vi "Facade.vi"(0 "Data In":T37={"Waveform"={"Type"=enum."Tone", "Tone"={"Frequency (kHz)"=0.0, "Phase (cycles)"=0.0, "Random phase"=FALSE}, "Pulse Train"={"Pulse width (us)"=0.0, "Pulse rate (Hz)"=0.0, "Gap (ms)"=0.0, "Polarity"=enum."POS", "PT State"={"Template"=[], "Nperiod"=0, "Index"=0, "Pulse Rate (Hz)"=0.0, "Phase (cycles)"=0.0, "Noff"=0}, "Asynch"=FALSE}, "Noise"={"Properties"={"InvFilt"=FALSE, "Aweight"=FALSE, "Seed"=0, "Tokens"=0, "Brickwall"=FALSE}, "Data"={"TokenNum"=0}}, "File"={"Filename"=path "", "Signal"=[], "Channel"=0, "stream"=FALSE, "offset"=0, "nreps"=0, "loops"=0, "Randomize"=FALSE, "order"=[], "Seed"=0, "Tokens"=0}, "FMSweep"={"Rate (oct/s)"=0.0, "Fmin (Hz)"=0.0, "Fmax (Hz)"=0.0, "Ramp (ms)"=0.0, "Linear"=FALSE}, "Chirp Train"={"Params"={"Fmin (kHz)"=4.0, "Fmax (kHz)"=64.0, "Compensate"=FALSE, "Duration (ms)"=2.0}, "Data"={"WF"=[]}}, "Complex Tone"={"Params"={"F0 (Hz)"=0.0, "Band"={"Flow (Hz)"=0.0, "Fhigh (Hz)"=0.0}, "Phase"=enum."Cosine", "Min F0 (Hz)"=0.0, "Max F0 (Hz)"=0.0, "ContinRandPhase"=FALSE, "Max peak factor"=inf, "Max mod depth"=2.0, "MinHarmNum"=0, "MaxHarmNum"=0, "Level Mode"=enum."per component", "% jitter"=0.0}, "Data"={"Ncomp"=0, "MinHarm"=0, "Phase"=[], "Amplitude"=[], "Npts/frame"=0, "Last F0"=0.0, "Fmin"=0.0, "Fmax"=0.0, "Lslope"=0.0, "randphase"=FALSE, "overall rms"=FALSE, "fmult"=[], "jittered"=FALSE}}, "FM"={"Carrier (kHz)"=0.0, "ModRate (Hz)"=0.0, "Depth (Hz)"=0.0, "Phase (cycles)"=0.0}, "Vowel"={"Freqs"="", "Set level"=enum."Total", "Freq"=[], "weights"=[]}, "Ramp"={"Duration (ms)"=0.0}}, "Filter"={"Type"=enum."Lowpass", "CF (kHz)"=0.0, "BW (kHz)"=0.0, "Cascade"=FALSE, "Quadrature"=FALSE, "Scale Factor"=0.0, "Stages"=[], "Class"=enum."Elliptic", "Order"=0, "BWUnits"=enum."Linear"}, "Burst"={"Active"=FALSE, "Delay (ms)"=0.0, "Duration (ms)"=50.0, "Ramp (ms)"=5.0, "Rate (Hz)"=0.0, "Trepeat (ms)"=0.0, "Repeat"=FALSE}, "Level"={"Level"=0.0, "Units"=enum."dB atten", "Max"=0.0, "Data"={"Multiplier"=0.0, "Cal File"=path "", "Cal"={"Freq (Hz)"=[], "Mag (dB SPL)"=[], "Phase (deg)"=[]}, "audiogram"=path ""}}, "Name"="", "Advanced"={"AltPol"=FALSE, "Var"="", "Expr"=""}, "SAM"={"Active"=FALSE, "Frequency (Hz)"=0.0, "Depth"=0.0, "Init Phase (cycles)"=0.0, "phase (degrees)"=0.0, "Asynch"=FALSE}, "Destination"={"Name"="", "Num"=0}} {"Filter"."Stages"."IIR Filter"."Forward Coefficients" format="%.4f"; "Filter"."Stages"."IIR Filter"."Reverse Coefficients" format="%.4f"}, 2 "Display State In":T29, 3 "Container State":T36) -> (6 "Data Out":T37={"Waveform"={"Type"=enum."Tone", "Tone"={"Frequency (kHz)"=0.0, "Phase (cycles)"=0.0, "Random phase"=FALSE}, "Pulse Train"={"Pulse width (us)"=0.0, "Pulse rate (Hz)"=0.0, "Gap (ms)"=0.0, "Polarity"=enum."POS", "PT State"={"Template"=[], "Nperiod"=0, "Index"=0, "Pulse Rate (Hz)"=0.0, "Phase (cycles)"=0.0, "Noff"=0}, "Asynch"=FALSE}, "Noise"={"Properties"={"InvFilt"=FALSE, "Aweight"=FALSE, "Seed"=0, "Tokens"=0, "Brickwall"=FALSE}, "Data"={"TokenNum"=0}}, "File"={"Filename"=path "", "Signal"=[], "Channel"=0, "stream"=FALSE, "offset"=0, "nreps"=0, "loops"=0, "Randomize"=FALSE, "order"=[], "Seed"=0, "Tokens"=0}, "FMSweep"={"Rate (oct/s)"=0.0, "Fmin (Hz)"=0.0, "Fmax (Hz)"=0.0, "Ramp (ms)"=0.0, "Linear"=FALSE}, "Chirp Train"={"Params"={"Fmin (kHz)"=4.0, "Fmax (kHz)"=64.0, "Compensate"=FALSE, "Duration (ms)"=2.0}, "Data"={"WF"=[]}}, "Complex Tone"={"Params"={"F0 (Hz)"=0.0, "Band"={"Flow (Hz)"=0.0, "Fhigh (Hz)"=0.0}, "Phase"=enum."Cosine", "Min F0 (Hz)"=0.0, "Max F0 (Hz)"=0.0, "ContinRandPhase"=FALSE, "Max peak factor"=inf, "Max mod depth"=2.0, "MinHarmNum"=0, "MaxHarmNum"=0, "Level Mode"=enum."per component", "% jitter"=0.0}, "Data"={"Ncomp"=0, "MinHarm"=0, "Phase"=[], "Amplitude"=[], "Npts/frame"=0, "Last F0"=0.0, "Fmin"=0.0, "Fmax"=0.0, "Lslope"=0.0, "randphase"=FALSE, "overall rms"=FALSE, "fmult"=[], "jittered"=FALSE}}, "FM"={"Carrier (kHz)"=0.0, "ModRate (Hz)"=0.0, "Depth (Hz)"=0.0, "Phase (cycles)"=0.0}, "Vowel"={"Freqs"="", "Set level"=enum."Total", "Freq"=[], "weights"=[]}, "Ramp"={"Duration (ms)"=0.0}}, "Filter"={"Type"=enum."Lowpass", "CF (kHz)"=0.0, "BW (kHz)"=0.0, "Cascade"=FALSE, "Quadrature"=FALSE, "Scale Factor"=0.0, "Stages"=[], "Class"=enum."Elliptic", "Order"=0, "BWUnits"=enum."Linear"}, "Burst"={"Active"=FALSE, "Delay (ms)"=0.0, "Duration (ms)"=50.0, "Ramp (ms)"=5.0, "Rate (Hz)"=0.0, "Trepeat (ms)"=0.0, "Repeat"=FALSE}, "Level"={"Level"=0.0, "Units"=enum."dB atten", "Max"=0.0, "Data"={"Multiplier"=0.0, "Cal File"=path "", "Cal"={"Freq (Hz)"=[], "Mag (dB SPL)"=[], "Phase (deg)"=[]}, "audiogram"=path ""}}, "Name"="", "Advanced"={"AltPol"=FALSE, "Var"="", "Expr"=""}, "SAM"={"Active"=FALSE, "Frequency (Hz)"=0.0, "Depth"=0.0, "Init Phase (cycles)"=0.0, "phase (degrees)"=0.0, "Asynch"=FALSE}, "Destination"={"Name"="", "Num"=0}} {"Filter"."Stages"."IIR Filter"."Forward Coefficients" format="%.4f"; "Filter"."Stages"."IIR Filter"."Reverse Coefficients" format="%.4f"}, 7 "Display State Out":T29, 8 "Action":T28)   [LabVIEW 2020, in "Stimulus Channel (G3).xctl"]
uses:
  Stimulus Channel (G3).xctl
  Full Stimulus Channel Data.ctl
  Waveform XControls/Waveform (G3)/Waveform Data.ctl
  Waveform VIs/Waveform Enum (V3).ctl
  Waveform XControls/Tone (G3)/Tone.Properties.ctl
  Waveform VIs/Pulse Train VIs/Pulse Train Params.ctl
  Waveform VIs/Pulse Train VIs/Pulse Polarity.ctl
  Waveform VIs/Pulse Train VIs/PT-Continuous State.ctl
  Waveform VIs/Noise VIs/Noise (G3).ctl
  Waveform VIs/Noise VIs/Noise (G3).Properties.ctl
  Waveform VIs/Noise VIs/Noise (G3).Data.ctl
  Waveform VIs/File VIs/StimFile-Params.ctl
  Waveform VIs/FM Sweep VIs/FM Sweep Params.ctl
  Waveform VIs/Chirp Train VIs/Chirp Train.ctl
  Waveform VIs/Chirp Train VIs/Chirp Train Params.ctl
  Waveform VIs/Complex Tone VIs/CT-Params.ctl
  Waveform VIs/Complex Tone VIs/CT-Phase Enum.ctl
  Waveform VIs/Complex Tone VIs/CT-Runtime Data.ctl
  Waveform XControls/FM Tone/Data.ctl
  Waveform XControls/Vowel/Vowel.Properties.ctl
  Waveform VIs/Ramp VIs/Ramp.Properties.ctl
  Filter (G3)/Filter Data.ctl
  Filter (G3)/Filter Type.ctl
  Filter VIs/Filter-Bandwidth Units.ctl
  Controls/Burst XCtl/Burst Data.ctl
  Level (G3)/Level Data.ctl
  Level (G3)/Level Units (G3).ctl
  Advanced Options (G3)/Advanced Options (G3).ctl
  Modulation VIs/SAM VIs/SAM Params.ctl
  Typedefs/Destination.ctl
  <vilib>/_xctls/Container State.ctl
  State.ctl
  Burst (G3)/Controls.ctl
  Waveform XControls/Waveform (G3)/Waveform (G3).xctl
  Level (G3)/Level (G3).xctl
  Utility VIs/Controls/KRing/KRing.xctl
  Burst (G3)/Burst (G3).xctl
  Waveform XControls/Waveform (G3)/Waveform (G3) - Persistent.ctl
  Waveform XControls/Noise (G3)/Noise (G3) - Persistent.ctl
  Calibration VIs/Endpoint VIs/LV Source/Endpoint-Spec.ctl
  Calibration VIs/Endpoint VIs/LV Source/Endpoint-Modality.ctl
  Calibration VIs/Endpoint VIs/LV Source/Endpoint-Laterality.ctl
  <vilib>/_xctls/Action.ctl
  Filter (G3)/Filter (G3).xctl
  Advanced Options (G3)/Advanced Options (G3).xctl
  <vilib>/_xctls/XControlSupport.lvlib
  Controls/Burst XCtl/Burst Control.xctl
  Waveform XControls/Noise (G3)/Noise (G3).xctl
  Waveform XControls/Tone (G3)/Tone (G3).xctl
  Waveform XControls/FM Tone/FM Tone.xctl
  Waveform XControls/Vowel/Vowel.xctl
panel:
  in  "display state signal":bool
  in  "Level Tab":enum32{"Level"}(tab)
  in  "Level":T2(xcontrol)
  in  "Tab Control 2":enum32{"Waveform"}(tab)
  in  "Waveform (G3)":T21(xcontrol)
  in  "Name":string
  in  "Destination":i16(xcontrol)
  in  "Tab Control":enum32{"Gate", "Modulation", "Filter", "More"}(tab)
  in  "Gate":T22(xcontrol)
  in  "SAM":T23
  in  "Filter":T26(xcontrol)
  in  "Advanced":T27(xcontrol)
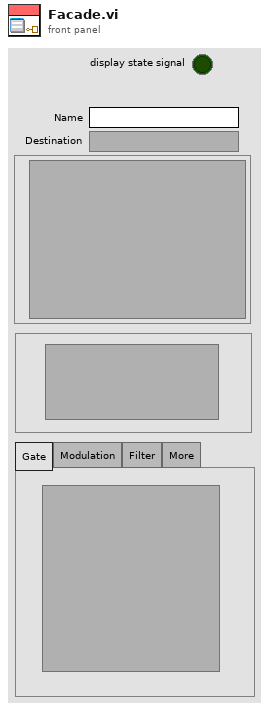
[diagram p1: front panel]
types:
  T1 = typedef "Level (G3).xctl/Level Units (G3).ctl" = enum16{"dB atten", "dB SPL", "dB re 1 Vrms", "dB V/Hz½", "mW", "dB HL", "Volts", "dB mW"}
  T2 = cluster{"Level":dbl, "Units":T1, "Max":dbl, "Data":cluster{"Multiplier":dbl, "Cal File":path, "Cal":cluster{"Freq (Hz)":dbl[], "Mag (dB SPL)":dbl[], "Phase (deg)":dbl[]}, "audiogram":path}}
  T3 = typedef "Waveform Enum (V3).ctl" = enum16{"OFF", "Tone", "Noise", "Pulse Train", "File", "FM Sweep", "Chirp Train", "Complex Tone", "FM Tone", "Vowel", "Ramp"}
  T4 = typedef "Tone (G3).xctl/Tone.Properties.ctl" = cluster{"Frequency (kHz)":dbl, "Phase (cycles)":dbl, "Random phase":bool}
  T5 = typedef "Pulse Train Params.ctl" = cluster{"Pulse width (us)":dbl, "Pulse rate (Hz)":dbl, "Gap (ms)":dbl, "Polarity":T6, "PT State":T7, "Asynch":bool}
  T6 = typedef "Pulse Polarity.ctl" = enum16{"POS", "NEG", "POS-NEG", "NEG-POS"}
  T7 = typedef "PT-Continuous State.ctl" = cluster{"Template":dbl[], "Nperiod":i32, "Index":i32, "Pulse Rate (Hz)":dbl, "Phase (cycles)":dbl, "Noff":i32}
  T8 = typedef "Noise (G3).ctl" = cluster{"Properties":T9, "Data":T10}
  T9 = typedef "Noise (G3).Properties.ctl" = cluster{"InvFilt":bool, "Aweight":bool, "Seed":i32, "Tokens":i32, "Brickwall":bool}
  T10 = typedef "Noise (G3).Data.ctl" = cluster{"TokenNum":i32}
  T11 = typedef "StimFile-Params.ctl" = cluster{"Filename":path, "Signal":dbl[], "Channel":i32, "stream":bool, "offset":i32, "nreps":i32, "loops":i32, "Randomize":bool, "order":i32[], "Seed":i32, "Tokens":i32}
  T12 = typedef "FM Sweep Params.ctl" = cluster{"Rate (oct/s)":dbl, "Fmin (Hz)":dbl, "Fmax (Hz)":dbl, "Ramp (ms)":dbl, "Linear":bool}
  T13 = typedef "Chirp Train.ctl" = cluster{"Params":T14, "Data":cluster{"WF":dbl[]}}
  T14 = typedef "Chirp Train Params.ctl" = cluster{"Fmin (kHz)":dbl, "Fmax (kHz)":dbl, "Compensate":bool, "Duration (ms)":dbl}
  T15 = typedef "CT-Params.ctl" = cluster{"F0 (Hz)":dbl, "Band":cluster{"Flow (Hz)":dbl, "Fhigh (Hz)":dbl}, "Phase":T16, "Min F0 (Hz)":dbl, "Max F0 (Hz)":dbl, "ContinRandPhase":bool, "Max peak factor":dbl, "Max mod depth":dbl, "MinHarmNum":i32, "MaxHarmNum":i32, "Level Mode":enum16{"per component", "overall rms"}, "% jitter":dbl}
  T16 = typedef "CT-Phase Enum.ctl" = enum16{"Cosine", "Random", "Alternating"}
  T17 = typedef "CT-Runtime Data.ctl" = cluster{"Ncomp":i32, "MinHarm":i32, "Phase":dbl[], "Amplitude":dbl[], "Npts/frame":i32, "Last F0":dbl, "Fmin":dbl, "Fmax":dbl, "Lslope":dbl, "randphase":bool, "overall rms":bool, "fmult":dbl[], "jittered":bool}
  T18 = typedef "FM Tone.xctl/Data.ctl" = cluster{"Carrier (kHz)":dbl, "ModRate (Hz)":dbl, "Depth (Hz)":dbl, "Phase (cycles)":dbl}
  T19 = typedef "Vowel.xctl/Vowel.Properties.ctl" = cluster{"Freqs":string, "Set level":enum16{"Total", "Per component"}, "Freq":dbl[], "weights":dbl[]}
  T20 = typedef "Ramp.Properties.ctl" = cluster{"Duration (ms)":dbl}
  T21 = cluster{"Type":T3, "Tone":T4, "Pulse Train":T5, "Noise":T8, "File":T11, "FMSweep":T12, "Chirp Train":T13, "Complex Tone":cluster{"Params":T15, "Data":T17}, "FM":T18, "Vowel":T19, "Ramp":T20}
  T22 = cluster{"Active":bool, "Delay (ms)":dbl, "Duration (ms)":dbl, "Ramp (ms)":dbl, "Rate (Hz)":dbl, "Trepeat (ms)":dbl, "Repeat":bool}
  T23 = cluster{"Active":bool, "Frequency (Hz)":dbl, "Depth (0-1)":dbl, "Phase (cycles)":dbl, "phase":dbl, "Asynch":bool}
  T24 = typedef "Filter (G3).xctl/Filter Type.ctl" = enum16{"OFF", "Lowpass", "Highpass", "Bandpass", "Bandstop"}
  T25 = typedef "Filter-Bandwidth Units.ctl" = enum16{"Linear", "Octaves", "Min-Max"}
  T26 = cluster{"Type":T24, "CF (kHz)":dbl, "BW (kHz)":dbl, "Cascade":bool, "Quadrature":bool, "Scale Factor":dbl, "Stages":cluster{"IIR Filter":cluster{"filter structure":enum32{"IIR 2nd Order", "IIR 4th Order"}, "Reverse Coefficients":dbl[], "Forward Coefficients":dbl[]}, "State":dbl[]}[], "Class":enum16{"Elliptic", "Butterworth"}, "Order":i32, "BWUnits":T25}
  T27 = cluster{"AltPol":bool, "Var":string, "Expr":string}
  T28 = typedef "XControlSupport.lvlib/Action.ctl" = cluster{"Data Changed?":bool, "State Changed?":bool, "Action Name":string}
  T29 = typedef "Stimulus Channel (G3).xctl/State.ctl" = cluster{"Show advanced":bool, "Show rove":bool, "Show name":bool, "Show dest":bool, "Lock dest":bool, "max level":dbl, "LMax Event":refnum<user-event>, "Controls":T30, "Level units":T1[], "Waveforms":T3[], "waveform":T31, "Endpoint Config":T33[], "multi":bool}
  T30 = typedef "Controls.ctl" = cluster{"Waveform":refnum<vi>, "Level":refnum<vi>, "Dest":refnum<vi>, "Gate":refnum<vi>}
  T31 = typedef "Waveform (G3).xctl/Waveform (G3) - Persistent.ctl" = cluster{"noise":T32, "Sort":bool}
  T32 = typedef "Noise (G3).xctl/Noise (G3) - Persistent.ctl" = cluster{"Show Aweight":bool}
  T33 = typedef "Endpoint-Spec.ctl" = cluster{"Name":string, "Modality":T34, "Laterality":T35, "CalFile":path, "Audiogram":path, "reuse cal?":bool}
  T34 = typedef "Endpoint-Modality.ctl" = enum16{"Unspecified", "Acoustic", "Electric", "Optical"}
  T35 = typedef "Endpoint-Laterality.ctl" = enum16{"N/A", "Right", "Left"}
  T36 = typedef "XControlSupport.lvlib/Container State.ctl" = cluster{"Indicator?":bool, "Run Mode?":bool, " Refnum":refnum<vi>}
  T37 = typedef "Stimulus Channel (G3).xctl/Full Stimulus Channel Data.ctl" = cluster{"Waveform":T38, "Filter":T39, "Burst":T40, "Level":T41, "Name":string, "Advanced":T42, "SAM":T43, "Destination":T44}
  T38 = typedef "Waveform (G3).xctl/Waveform Data.ctl" = cluster{"Type":T3, "Tone":T4, "Pulse Train":T5, "Noise":T8, "File":T11, "FMSweep":T12, "Chirp Train":T13, "Complex Tone":cluster{"Params":T15, "Data":T17}, "FM":T18, "Vowel":T19, "Ramp":T20}
  T39 = typedef "Filter (G3).xctl/Filter Data.ctl" = cluster{"Type":T24, "CF (kHz)":dbl, "BW (kHz)":dbl, "Cascade":bool, "Quadrature":bool, "Scale Factor":dbl, "Stages":cluster{"IIR Filter":cluster{"filter structure":enum32{"IIR 2nd Order", "IIR 4th Order"}, "Reverse Coefficients":dbl[], "Forward Coefficients":dbl[]}, "State":dbl[]}[], "Class":enum16{"Elliptic", "Butterworth"}, "Order":i32, "BWUnits":T25}
  T40 = typedef "Burst Control.xctl/Burst Data.ctl" = cluster{"Active":bool, "Delay (ms)":dbl, "Duration (ms)":dbl, "Ramp (ms)":dbl, "Rate (Hz)":dbl, "Trepeat (ms)":dbl, "Repeat":bool}
  T41 = typedef "Level (G3).xctl/Level Data.ctl" = cluster{"Level":dbl, "Units":T1, "Max":dbl, "Data":cluster{"Multiplier":dbl, "Cal File":path, "Cal":cluster{"Freq (Hz)":dbl[], "Mag (dB SPL)":dbl[], "Phase (deg)":dbl[]}, "audiogram":path}}
  T42 = typedef "Advanced Options (G3).xctl/Advanced Options (G3).ctl" = cluster{"AltPol":bool, "Var":string, "Expr":string}
  T43 = typedef "SAM Params.ctl" = cluster{"Active":bool, "Frequency (Hz)":dbl, "Depth":dbl, "Init Phase (cycles)":dbl, "phase (degrees)":dbl, "Asynch":bool}
  T44 = typedef "Destination.ctl" = cluster{"Name":string, "Num":i32}
  T45 = enum8{"Enabled", "Disabled", "Disabled and Grayed Out"}
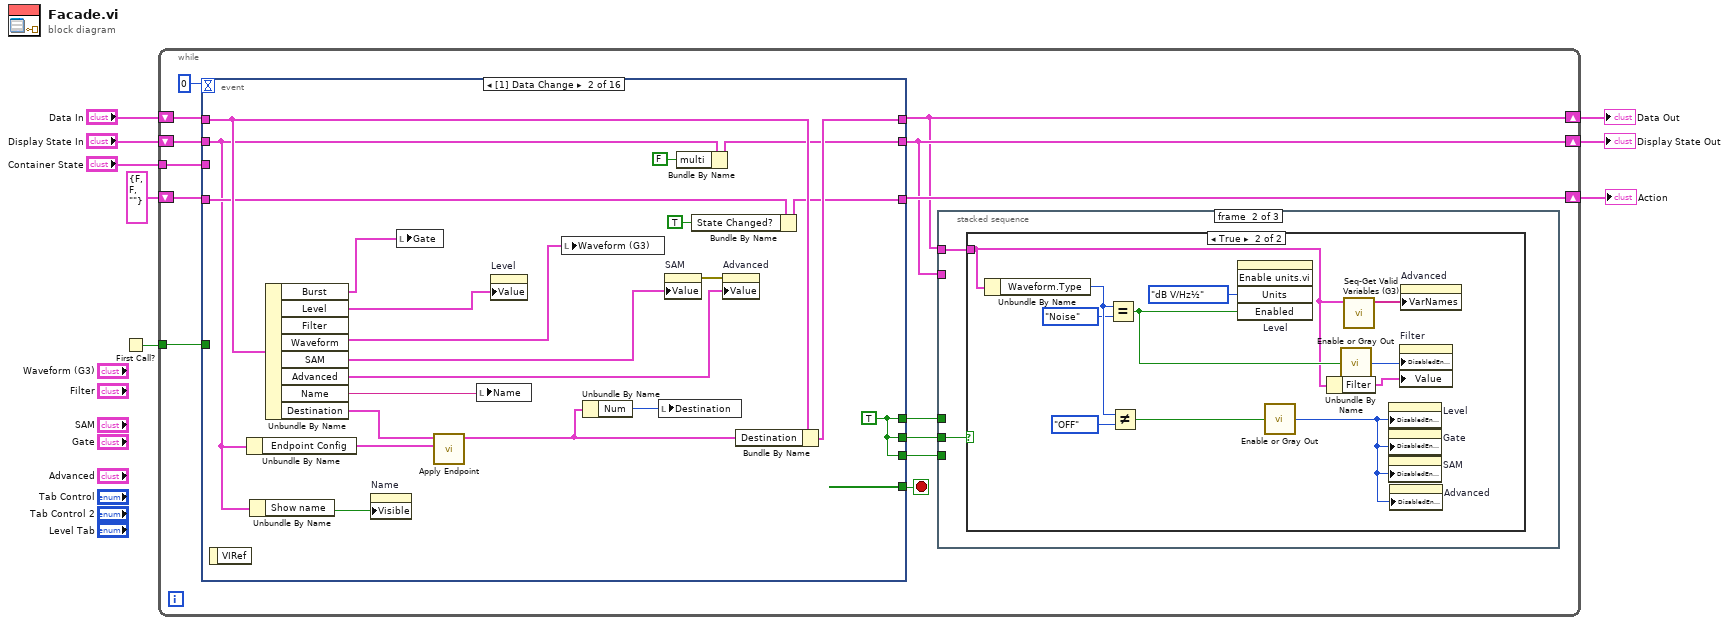
[diagram p0: block diagram]
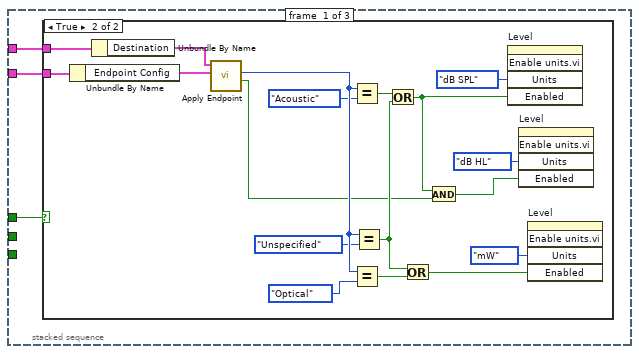
[diagram p2: hidden frame]
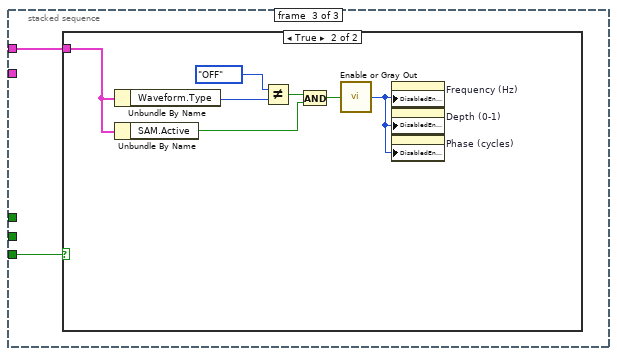
[diagram p5: hidden frame]
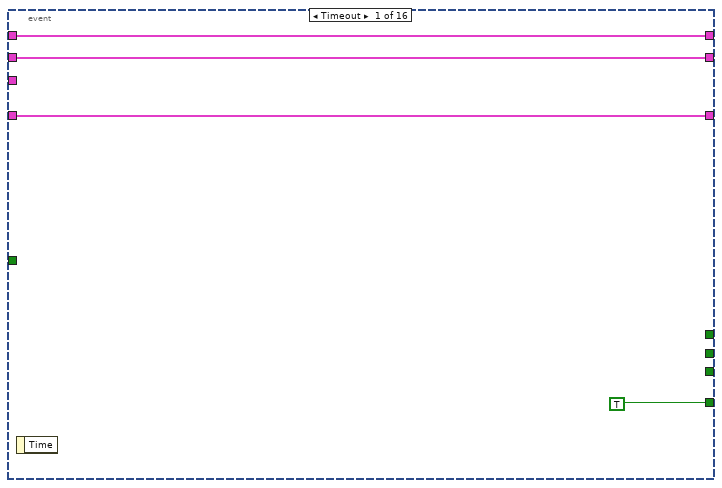
[diagram p7: hidden frame]
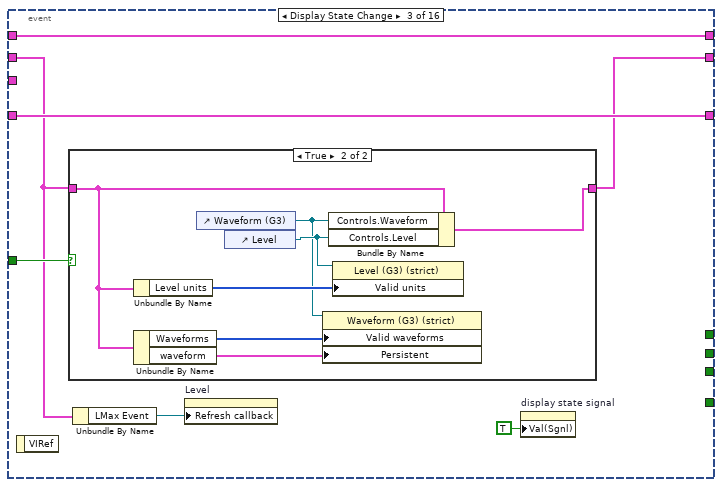
[diagram p8: hidden frame]
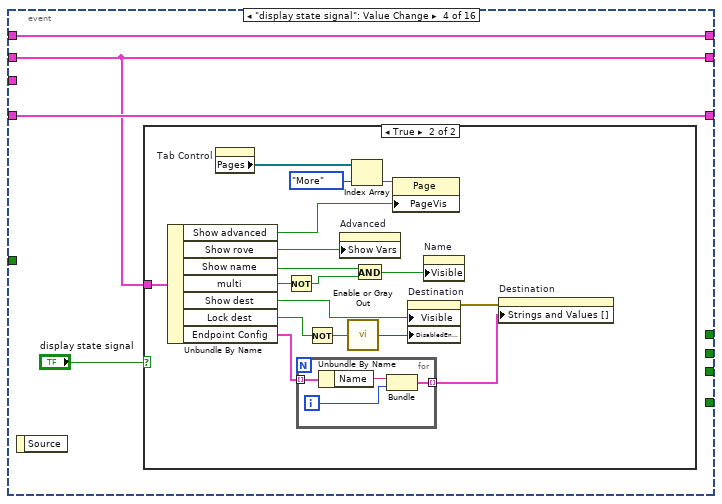
[diagram p10: hidden frame]
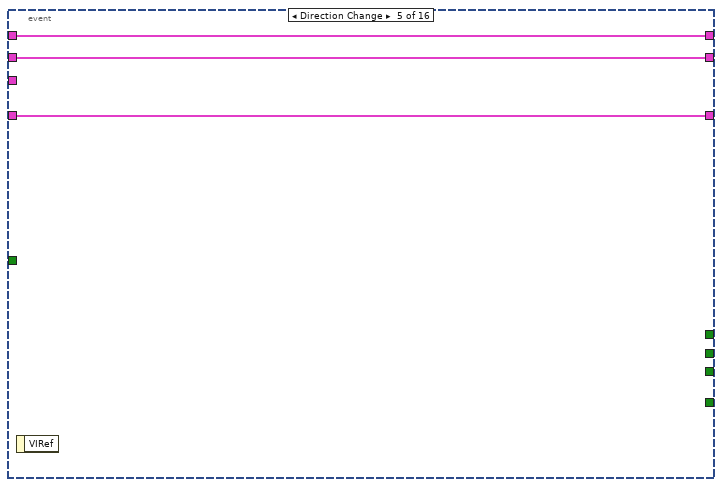
[diagram p12: hidden frame]
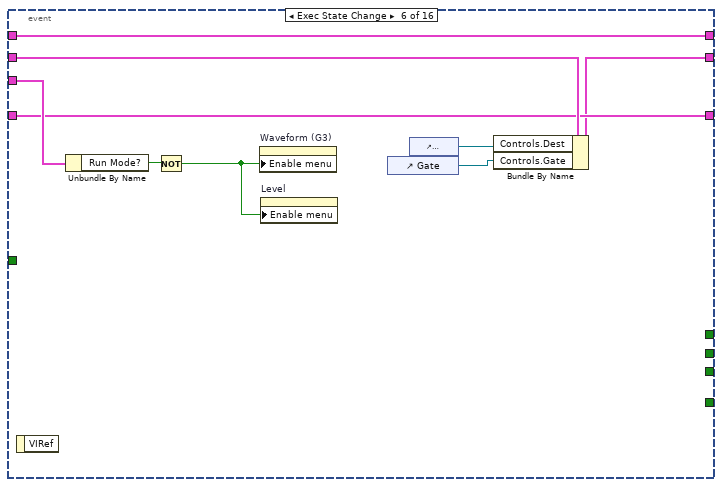
[diagram p13: hidden frame]
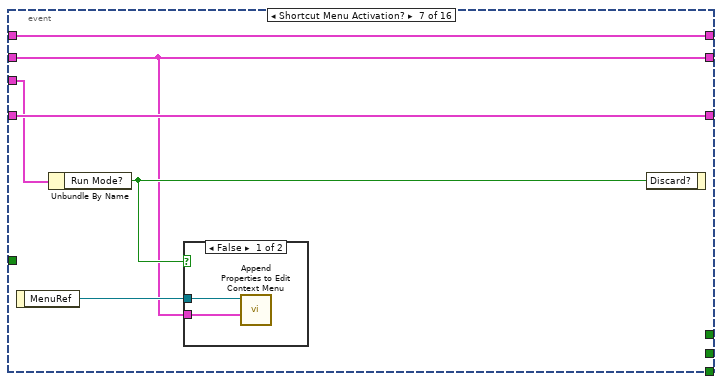
[diagram p14: hidden frame]
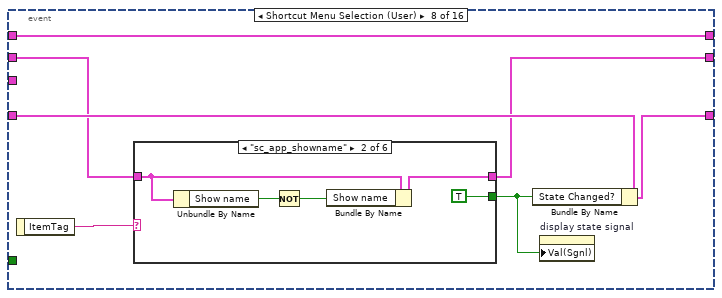
[diagram p16: hidden frame]
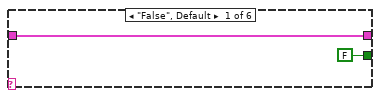
[diagram p17: hidden frame]
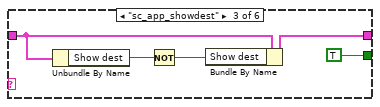
[diagram p18: hidden frame]
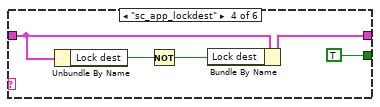
[diagram p19: hidden frame]
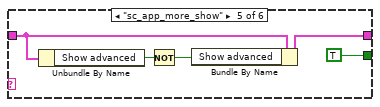
[diagram p20: hidden frame]
diagram:
  n1 = First Call?() -> (First Call?: T/F=w1:bool)
  n2 = while {
    shift-right: [w12] -> w5
    shift-left: "Display State In" -> [w21]
    tunnel: "Container State" -> [w19]
    shift-right: [w11] -> w8
    shift-left: "Data In" -> [w18]
    shift-right: [w16] -> w3
    shift-left: T28 {"Data Changed?"=FALSE, "State Changed?"=FALSE, "Action Name"=""} ("Action") -> [w17]
    tunnel: w1 -> [w14]
    stop <- w20 stop-if-true
    n3 = event shown="[1] Data Change" {
      selector: _ -> [_ _ _ _ _ _ _ _ _ _ _ _ _ _ _ _]
      dyn-events: _ -> [_ _ _ _ _ _ _ _ _ _ _ _ _ _ _ _]
      timeout: 0 -> [_ _ _ _ _ _ _ _ _ _ _ _ _ _ _ _]
      tunnel: w21 -> [w65 w75 w92 w106 w132 w140 w142 w153 w190 w193 w216 w226 w237 w241 w252 w258]
      tunnel: [w65 w72 w93 w106 w132 w135 w142 w152 w190 w193 w209 w226 w237 w241 w246 w258] -> w12
      tunnel: [TRUE _ _ _ _ _ _ _ _ _ _ _ _ _ _ _] -> w20
      tunnel: w19 -> [_ _ _ _ _ w141 w145 _ _ _ _ _ _ _ _ _]
      tunnel: w18 -> [w66 w89 w96 w108 w131 w139 w147 w156 w189 w201 w211 w225 w231 w240 w251 w257]
      tunnel: [w66 w87 w96 w108 w131 w139 w147 w156 w185 w198 w206 w224 w235 w239 w249 w256] -> w11
      tunnel: [w67 w77 w95 w107 w130 w138 w146 w154 w187 w199 w217 w227 w234 w242 w253 w259] -> w16
      tunnel: w17 -> [w67 w88 w95 w107 w130 w138 w146 w155 w188 w200 w218 w229 w236 w244 w254 w261]
      tunnel: w14 -> [_ _ w94 _ _ _ _ _ _ _ _ _ _ _ _ _]
      tunnel: [_ w86 _ _ _ _ _ _ _ TRUE ("Value (Signaling)") _ _ _ _ _ _] -> w13
      tunnel: [_ w86 _ _ _ _ _ _ _ _ TRUE ("Value (Signaling)") _ _ _ _ _] -> w10
      tunnel: [_ w86 _ _ _ _ _ _ _ _ _ _ TRUE ("Value (Signaling)") _ _ _] -> w9
      event Timeout {
        n4 = event-data() -> ()  [unwired: 1 in, 1 out]
      }
      event Data Change {
        w86 = TRUE ("Value (Signaling)")
        n5 = event-data() -> ()  [unwired: 1 in, 1 out]
        n6 = Unbundle By Name(w75) -> ("Endpoint Config"=w82:T33[])
        n7 = Unbundle By Name(w75) -> ("Show name"=w74:bool)
        n8 = Unbundle By Name(w89) -> ("Burst"=w70:T40, "Level"=w69:T41, "Waveform"=w73:T38, "SAM"=w85:T43, "Advanced"=w84:T42, "Name"=w83:string, "Destination"=w81:T44)  [unwired: 1 out]
        n9 = property on="Name" class="Str"("Visible"=w74) -> ()  [unwired: 2 in, 2 out]
        n10 = local write "Gate"(w70) -> ()
        n11 = call "Apply Endpoint.vi"("Endpoint Config"=w82, "Destination In"=w81) -> ("Destination Out"=w80:T44)  [unwired: 7 in, 2 out]
        n12 = local write "Name"(w83) -> ()
        n13 = property on="Level" class="Level (G3) (strict)"("Value"=w69) -> ()  [unwired: 2 in, 2 out]
        n14 = local write "Waveform (G3)"(w73) -> ()
        n15 = Unbundle By Name(w80) -> ("Num"=w79:i32)
        n16 = local write "Destination"(w79) -> ()
        n17 = property on="SAM" class="Clust (strict)"("Value"=w85) -> (error out=w78:errorcluster)  [unwired: 2 in, 1 out]
        n18 = Bundle By Name(cluster=w75, "multi"=FALSE) -> (w72:T29)
        n19 = Bundle By Name(cluster=w88, "State Changed?"=TRUE) -> (w77:T28)
        n20 = property on="Advanced" class="Advanced Options (G3) (strict)"(error in=w78, "Value"=w84) -> ()  [unwired: 1 in, 2 out]
        n21 = Bundle By Name(cluster=w89, "Destination"=w80) -> (w87:T37)
      }
      event Display State Change {
        n22 = event-data() -> ()  [unwired: 1 in, 1 out]
        n23 = case shown="True" w94 {
          tunnel: w92 -> [w97 w103]
          tunnel: [w97 w104] -> w93
          frame False {
          }
          frame True {
            n24 = Unbundle By Name(w103) -> ("Level units"=w101:T1[])
            n25 = Unbundle By Name(w103) -> ("Waveforms"=w100:T3[], "waveform"=w99:T31)
            n26 = control-ref of="Waveform (G3)"() -> (w98:refnum<vi>)
            n27 = control-ref of="Level"() -> (w102:refnum<vi>)
            n28 = property class="Waveform (G3) (strict)"(reference=w98, "Valid waveforms"=w100, "Persistent"=w99) -> ()  [unwired: 1 in, 2 out]
            n29 = Bundle By Name(cluster=w103, "Controls.Waveform"=w98, "Controls.Level"=w102) -> (w104:T29)
            n30 = property class="Level (G3) (strict)"(reference=w102, "Valid units"=w101) -> ()  [unwired: 1 in, 2 out]
          }
        }
        n31 = Unbundle By Name(w92) -> ("LMax Event"=w91:refnum<user-event>)
        n32 = property on="Level" class="Level (G3) (strict)"("Refresh callback"=w91) -> ()  [unwired: 2 in, 2 out]
        n33 = property on="display state signal" class="Bool (strict)"("Val(Sgnl)"=TRUE ("Value (Signaling)")) -> ()  [unwired: 2 in, 2 out]
      }
      event "display state signal": Value Change {
        n34 = event-data() -> ()  [unwired: 1 in, 1 out]
        n35 = case shown="True" "display state signal" {
          tunnel: w106 -> [_ w125]
          frame False {
          }
          frame True {
            n36 = Unbundle By Name(w125) -> ("Show advanced"=w122:bool, "Show rove"=w120:bool, "Show name"=w112:bool, "multi"=w111:bool, "Show dest"=w119:bool, "Lock dest"=w117:bool, "Endpoint Config"=w116:T33[])
            n37 = property on="Tab Control" class="TabCtl (strict)"() -> ("Pages"=w124:refnum<vi>[])  [unwired: 2 in, 2 out]
            n38 = Not(x=w111) -> (.not. x?=w110:bool)
            n39 = for {
              tunnel: w116 -> [w129] mode=indexing
              tunnel: [w127] -> w113 mode=indexing
              i -> [w126]
              n40 = Unbundle By Name(w129) -> ("Name"=w128:string)
              n41 = Bundle("Name"=w128, w126) -> (w127:cluster{"Name":string, i32})  [unwired: 1 in]
            }
            n42 = Not(x=w117) -> (.not. x?=w118:bool)
            n43 = property on="Advanced" class="Advanced Options (G3) (strict)"("Show Vars"=w120) -> ()  [unwired: 2 in, 2 out]
            n44 = call "Enable or Gray Out.vi"("Boolean"=w118) -> ("Disabled"=w115:T45)
            n45 = Index Array(array=w124, index=enum32{"Gate", "Modulation", "Filter", "More"}."More" ("Tab Control")) -> (element=w123:refnum<vi>)
            n46 = And(x=w112, y=w110) -> (x .and. y?=w109:bool)
            n47 = property class="Page"(reference=w123, "PageVis"=w122) -> ()  [unwired: 1 in, 2 out]
            n48 = property on="Destination" class="KRing (strict)"("Visible"=w119, "DisabledEnum"=w115) -> (error out=w114:errorcluster)  [unwired: 2 in, 1 out]
            n49 = property on="Name" class="Str"("Visible"=w109) -> ()  [unwired: 2 in, 2 out]
            n50 = property on="Destination" class="KRing (strict)"(error in=w114, "Strings and Values []"=w113) -> ()  [unwired: 1 in, 2 out]
          }
        }
      }
      event Direction Change {
        n51 = event-data() -> ()  [unwired: 1 in, 1 out]
      }
      event Exec State Change {
        n52 = event-data() -> ()  [unwired: 1 in, 1 out]
        n53 = Unbundle By Name(w141) -> ("Run Mode?"=w137:bool)
        n54 = Not(x=w137) -> (.not. x?=w136:bool)
        n55 = property on="Waveform (G3)" class="Waveform (G3) (strict)"("Enable menu"=w136) -> ()  [unwired: 2 in, 2 out]
        n56 = property on="Level" class="Level (G3) (strict)"("Enable menu"=w136) -> ()  [unwired: 2 in, 2 out]
        n57 = control-ref of="Gate"() -> (w133:refnum<vi>)
        n58 = control-ref of="Destination"() -> (w134:refnum<vi>)
        n59 = Bundle By Name(cluster=w140, "Controls.Dest"=w134, "Controls.Gate"=w133) -> (w135:T29)
      }
      event Shortcut Menu Activation? {
        n60 = event-data() -> ("MenuRef"=w144:refnum<k9>)  [unwired: 1 in]
        n61 = Unbundle By Name(w145) -> ("Run Mode?"=w143:bool)
        n62 = case shown="False" w143 {
          tunnel: w144 -> [w149 _]
          tunnel: w142 -> [w148 _]
          frame False {
            n63 = call "Append Properties to Edit Context Menu.vi"("State"=w148, "Menu in"=w149) -> ()  [unwired: 10 in]
          }
          frame True {
          }
        }
        n64 = event-data("Discard?"=w143) -> ()  [unwired: 1 in, 1 out]
      }
      event Shortcut Menu Selection (User) {
        n65 = event-data() -> ("ItemTag"=w150:string)  [unwired: 1 in]
        n66 = case shown="\"sc_app_showname\"" w150 {
          tunnel: [w158 w163 w168 w173 w178 w183] -> w152
          tunnel: w153 -> [w158 w160 w165 w170 w175 w180]
          tunnel: [FALSE TRUE TRUE TRUE TRUE TRUE] -> w151
          frame "False", Default {
          }
          frame "sc_app_showname" {
            n67 = Unbundle By Name(w160) -> ("Show name"=w162:bool)
            n68 = Not(x=w162) -> (.not. x?=w161:bool)
            n69 = Bundle By Name(cluster=w160, "Show name"=w161) -> (w163:T29)
          }
          frame "sc_app_showdest" {
            n70 = Unbundle By Name(w165) -> ("Show dest"=w167:bool)
            n71 = Not(x=w167) -> (.not. x?=w166:bool)
            n72 = Bundle By Name(cluster=w165, "Show dest"=w166) -> (w168:T29)
          }
          frame "sc_app_lockdest" {
            n73 = Unbundle By Name(w170) -> ("Lock dest"=w172:bool)
            n74 = Not(x=w172) -> (.not. x?=w171:bool)
            n75 = Bundle By Name(cluster=w170, "Lock dest"=w171) -> (w173:T29)
          }
          frame "sc_app_more_show" {
            n76 = Unbundle By Name(w175) -> ("Show advanced"=w177:bool)
            n77 = Not(x=w177) -> (.not. x?=w176:bool)
            n78 = Bundle By Name(cluster=w175, "Show advanced"=w176) -> (w178:T29)
          }
          frame "sc_app_more_show_vars" {
            n79 = Unbundle By Name(w180) -> ("Show rove"=w182:bool)
            n80 = Not(x=w182) -> (.not. x?=w181:bool)
            n81 = Bundle By Name(cluster=w180, "Show rove"=w181) -> (w183:T29)
          }
        }
        n82 = Bundle By Name(cluster=w155, "State Changed?"=w151) -> (w154:T28)
        n83 = property on="display state signal" class="Bool (strict)"("Val(Sgnl)"=w151) -> ()  [unwired: 2 in, 2 out]
      }
      event "Name": Value Change {
        n84 = event-data() -> ()  [unwired: 1 in, 1 out]
        n85 = Bundle By Name(cluster=w188, "Data Changed?"=TRUE) -> (w187:T28)
        n86 = Bundle By Name(cluster=w189, "Name"="Name") -> (w185:T37)
      }
      event "Destination": Value Change {
        n87 = event-data() -> ()  [unwired: 1 in, 1 out]
        n88 = Unbundle By Name(w193) -> ("Endpoint Config"=w197:T33[])
        n89 = Index Array(array=w197, index="Destination") -> (element=w196:T33)
        n90 = Unbundle By Name(w196) -> ("Name"=w195:string)
        n91 = Bundle By Name(cluster=w201, "Destination.Name"=w195, "Destination.Num"="Destination") -> (w198:T37)
        n92 = Bundle By Name(cluster=w200, "Data Changed?"=TRUE) -> (w199:T28)
      }
      event "Waveform (G3)": Value Change {
        w210 = TRUE ("Data Changed?")
        n93 = event-data() -> ("NewVal"=w215:T21)  [unwired: 1 in]
        n94 = Unbundle By Name(w215) -> ("Type"=w212:T3)
        n95 = Unbundle By Name(w211) -> ("Filter.Type"=w213:T24)
        n96 = Equal?(x=w212, y=Waveform_Enum_(V3)."Noise") -> (x = y?=w205:bool)
        n97 = property on="Waveform (G3)" class="Waveform (G3) (strict)"() -> ("Valid waveforms"=w208:T3[], "Persistent"=w207:T31)  [unwired: 2 in, 2 out]
        n98 = Select(t=w213, s=w205, f=Filter_Type."OFF") -> (s? t:f=w204:T24)
        n99 = Bundle By Name(cluster=w216, "Waveforms"=w208, "waveform"=w207) -> (w209:T29)
        n100 = Bundle By Name(cluster=w211, "Waveform"=w215, "Filter.Type"=w204) -> (w206:T37)
        n101 = Bundle By Name(cluster=w218, "Data Changed?"=w210, "State Changed?"=w210) -> (w217:T28)
      }
      event "Filter": Value Change {
        n102 = event-data() -> ("NewVal.Type"=w221:T24, "NewVal.CF (kHz)"=w223:dbl, "NewVal.BW (kHz)"=w222:dbl, "NewVal.Cascade"=w220:bool, "NewVal.BWUnits"=w219:T25)  [unwired: 1 in]
        n103 = Bundle By Name(cluster=w225, "Filter.Type"=w221, "Filter.CF (kHz)"=w223, "Filter.BW (kHz)"=w222, "Filter.Cascade"=w220, "Filter.BWUnits"=w219) -> (w224:T37)
        n104 = Bundle By Name(cluster=w229, "Data Changed?"=TRUE) -> (w227:T28)
      }
      event "SAM": Value Change {
        n105 = event-data() -> ("NewVal"=w232:T23)  [unwired: 1 in]
        n106 = Bundle By Name(cluster=w231, "SAM"=w232) -> (w235:T37)
        n107 = Bundle By Name(cluster=w236, "Data Changed?"=TRUE) -> (w234:T28)
      }
      event "Gate": Value Change {
        n108 = event-data() -> ("NewVal"=w238:T22)  [unwired: 1 in]
        n109 = Bundle By Name(cluster=w240, "Burst"=w238) -> (w239:T37)
        n110 = Bundle By Name(cluster=w244, "Data Changed?"=TRUE) -> (w242:T28)
      }
      event "Level": Value Change {
        w247 = TRUE ("Data Changed?")
        n111 = event-data() -> ()  [unwired: 1 in, 1 out]
        n112 = Bundle By Name(cluster=w251, "Level"="Level") -> (w249:T37)
        n113 = property on="Level" class="Level (G3) (strict)"() -> ("Valid units"=w245:T1[])  [unwired: 2 in, 2 out]
        n114 = Bundle By Name(cluster=w254, "Data Changed?"=w247, "State Changed?"=w247) -> (w253:T28)
        n115 = Bundle By Name(cluster=w252, "Level units"=w245) -> (w246:T29)
        n116 = call "Seq-Get Valid Variables (G3).vi"("StimChan"=w249) -> ("VarNames"=w250:string[])  [unwired: 10 in]
        n117 = property on="Advanced" class="Advanced Options (G3) (strict)"("VarNames"=w250) -> ()  [unwired: 2 in, 2 out]
      }
      event "Advanced": Value Change {
        n118 = event-data() -> ("NewVal"=w255:T27)  [unwired: 1 in]
        n119 = Bundle By Name(cluster=w257, "Advanced"=w255) -> (w256:T37)
        n120 = Bundle By Name(cluster=w261, "Data Changed?"=TRUE) -> (w259:T28)
      }
    }
    n121 = stacked-sequence {
      tunnel: w13 -> [w24 _ _]
      tunnel: w12 -> [w23 _ _]
      tunnel: w11 -> [w22 w44 w57]
      tunnel: w10 -> [_ w43 _]
      tunnel: w9 -> [_ _ w56]
      frame #0 {
        n122 = case shown="True" w24 {
          tunnel: w23 -> [_ w30]
          tunnel: w22 -> [_ w29]
          frame False {
          }
          frame True {
            n123 = Unbundle By Name(w30) -> ("Endpoint Config"=w31:T33[])
            n124 = Unbundle By Name(w29) -> ("Destination"=w32:T44)
            n125 = call "Apply Endpoint.vi"("Endpoint Config"=w31, "Destination In"=w32) -> ("Have audiogram"=w36:bool, "Modality"=w39:T34)  [unwired: 7 in, 1 out]
            n126 = Equal?(x=w39, y=Endpoint-Modality."Acoustic") -> (x = y?=w37:bool)
            n127 = Equal?(x=w39, y=Endpoint-Modality."Optical") -> (x = y?=w34:bool)
            n128 = Equal?(x=w39, y=Endpoint-Modality."Unspecified") -> (x = y?=w42:bool)
            n129 = Or(x=w37, y=w42) -> (x .or. y?=w41:bool)
            n130 = Or(x=w42, y=w34) -> (x .or. y?=w40:bool)
            n131 = And(x=w41, y=w36) -> (x .and. y?=w28:bool)
            n132 = invoke on="Level" class="Level (G3) (strict)" method="Enable units.vi"("Units"=Level_Units_(G3)."dB SPL", "Enabled"=w41) -> ()  [unwired: 3 in, 5 out]
            n133 = invoke on="Level" class="Level (G3) (strict)" method="Enable units.vi"("Units"=Level_Units_(G3)."dB HL", "Enabled"=w28) -> ()  [unwired: 3 in, 5 out]
            n134 = invoke on="Level" class="Level (G3) (strict)" method="Enable units.vi"("Units"=Level_Units_(G3)."mW", "Enabled"=w40) -> ()  [unwired: 3 in, 5 out]
          }
        }
      }
      frame #1 {
        n135 = case shown="True" w43 {
          tunnel: w44 -> [_ w45]
          frame False {
          }
          frame True {
            n136 = Unbundle By Name(w45) -> ("Waveform.Type"=w47:T3)
            n137 = Equal?(x=w47, y=Waveform_Enum_(V3)."Noise") -> (x = y?=w55:bool)
            n138 = Not Equal?(x=w47, y=Waveform_Enum_(V3)."OFF") -> (x != y?=w51:bool)
            n139 = invoke on="Level" class="Level (G3) (strict)" method="Enable units.vi"("Units"=Level_Units_(G3)."dB V/Hz½", "Enabled"=w55) -> ()  [unwired: 3 in, 5 out]
            n140 = call "Enable or Gray Out.vi"("Boolean"=w51) -> ("Disabled"=w52:T45)
            n141 = Unbundle By Name(w45) -> ("Filter"=w54:T39)
            n142 = call "Enable or Gray Out.vi"("Boolean"=w55) -> ("Disabled"=w50:T45)
            n143 = call "Seq-Get Valid Variables (G3).vi"("StimChan"=w45) -> ("VarNames"=w49:string[])  [unwired: 10 in]
            n144 = property on="Level" class="Level (G3) (strict)"("DisabledEnum"=w52) -> ()  [unwired: 2 in, 2 out]
            n145 = property on="Gate" class="Burst (G3) (strict)"("DisabledEnum"=w52) -> ()  [unwired: 2 in, 2 out]
            n146 = property on="SAM" class="Clust (strict)"("DisabledEnum"=w52) -> ()  [unwired: 2 in, 2 out]
            n147 = property on="Advanced" class="Advanced Options (G3) (strict)"("DisabledEnum"=w52) -> ()  [unwired: 2 in, 2 out]
            n148 = property on="Filter" class="Filter (G3) (strict)"("DisabledEnum"=w50, "Value"=w54) -> ()  [unwired: 2 in, 2 out]
            n149 = property on="Advanced" class="Advanced Options (G3) (strict)"("VarNames"=w49) -> ()  [unwired: 2 in, 2 out]
          }
        }
      }
      frame #2 {
        n150 = case shown="True" w56 {
          tunnel: w57 -> [_ w58]
          frame False {
          }
          frame True {
            n151 = Unbundle By Name(w58) -> ("Waveform.Type"=w59:T3)
            n152 = Unbundle By Name(w58) -> ("SAM.Active"=w62:bool)
            n153 = Not Equal?(x=Waveform_Enum_(V3)."OFF", y=w59) -> (x != y?=w61:bool)
            n154 = And(x=w61, y=w62) -> (x .and. y?=w63:bool)
            n155 = call "Enable or Gray Out.vi"("Boolean"=w63) -> ("Disabled"=w64:T45)
            n156 = property on="Frequency (Hz)" class="DigNum (strict)"("DisabledEnum"=w64) -> ()  [unwired: 2 in, 2 out]
            n157 = property on="Depth (0-1)" class="DigNum (strict)"("DisabledEnum"=w64) -> ()  [unwired: 2 in, 2 out]
            n158 = property on="Phase (cycles)" class="DigNum (strict)"("DisabledEnum"=w64) -> ()  [unwired: 2 in, 2 out]
          }
        }
      }
    }
  }
  "Display State Out" <- w5
  "Data Out" <- w8
  "Action" <- w3
